vi "Video Playback.vi"() -> ()   [LabVIEW 2020, in "examples.lvlib"]
uses:
  examples.lvlib
  video_io/Reader/Reader.lvclass/Reader.ctl
  video_io/Reader/Reader.lvclass
  image/New Image (ARGB Preallocated).vi
  image/Size (ARGB).vi
  video_io/Reader/Set Frame Position (Index).vi
  video_io/Reader/Read Frame (ARGB Next).vi
  image/Draw Image to Picture (ARGB).vi
  video_io/Reader/Get Frame Position (Index).vi
  image/New Image (ARGB Preallocated).vi/3321fa97-f432-4e1e-8db9-a0df79aed21b.vi
  image/ARGB Colour to U32 Pixel Value.vi
  image/Size (ARGB).vi/69a1505b-b287-44ed-9ef9-f10ed7b260f4.vi
  video_io/Reader/Set Frame Position (Index).vi/acb2feee-aaa4-4f40-955f-c8ac8e9dff35.vi
  video_io/Reader/Read Frame (ARGB Next).vi/9eeb12df-7581-4bcd-a397-18dbd97d2298.vi
  image/Draw Image to Picture (ARGB).vi/8cd07b1b-062e-4fe4-9e87-2eb3dc89fe0e.vi
  video_io/Reader/Get Frame Position (Index).vi/acb2feee-aaa4-4f40-955f-c8ac8e9dff35.vi
  <vilib>/Utility/error.llb/Error Cluster From Error Code.vi
  image/image.lvlib
panel:
  out "File OK":bool
  in  "Play":bool
  in  "Video File":path
  in  "Position":u64(slide) scale=0.0..37.0
  out "Picture":picture
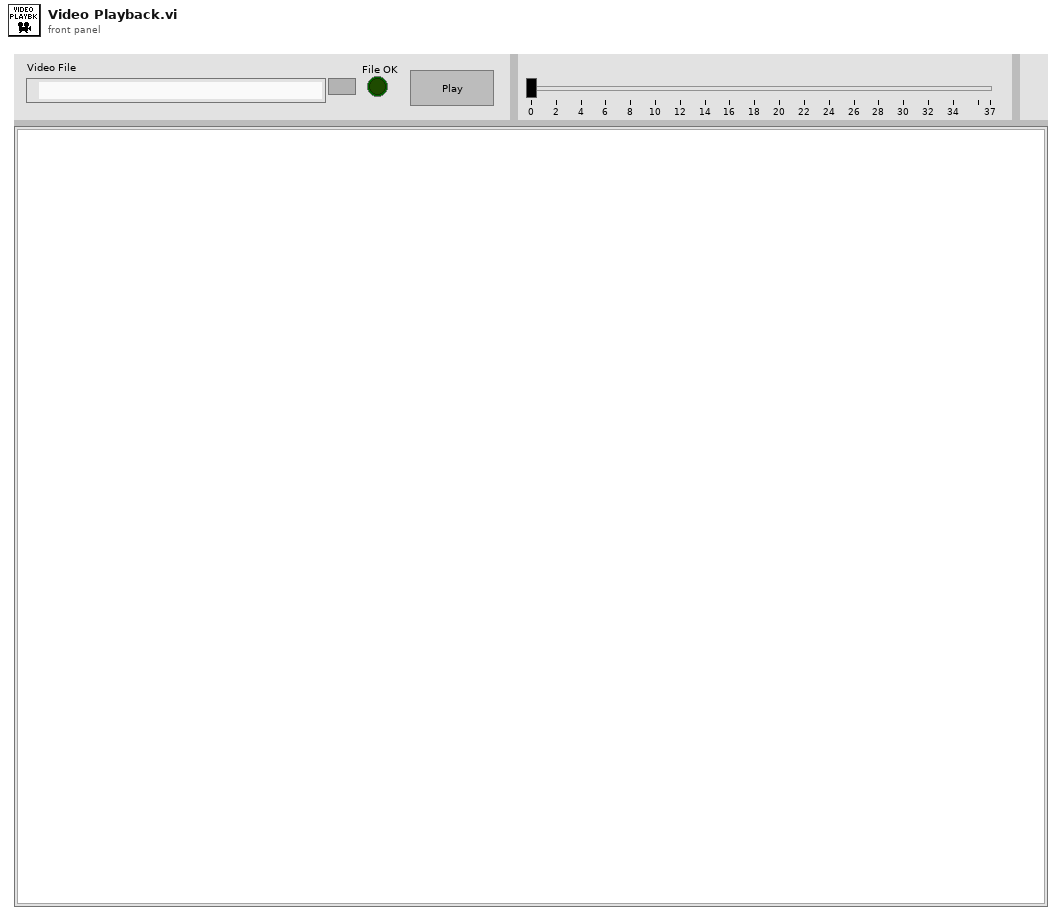
[diagram p1: front panel]
types:
  T1 = typedef "image.lvlib/ARGB Image.ctl" = refnum<data-value>
  T2 = enum8{"Enabled", "Disabled", "Disabled and Grayed Out"}
  T3 = typedef "common.lvlib/Image Size (Integer).ctl" = cluster{"Width":u16, "Height":u16}
  T4 = typedef "image.lvlib/Image Draw Offset.ctl" = cluster{"Left":i16, "Top":i16}
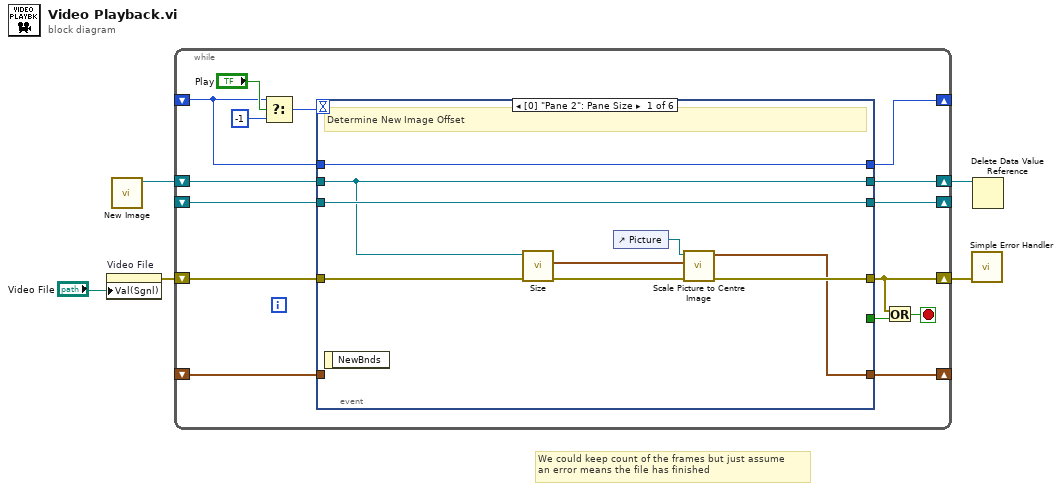
[diagram p0: block diagram]
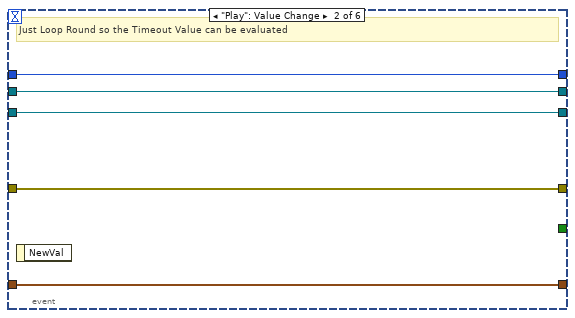
[diagram p2: hidden frame]
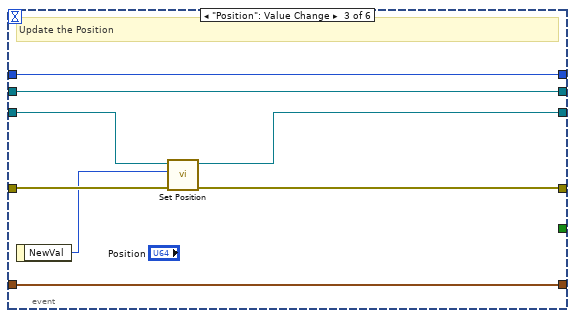
[diagram p3: hidden frame]
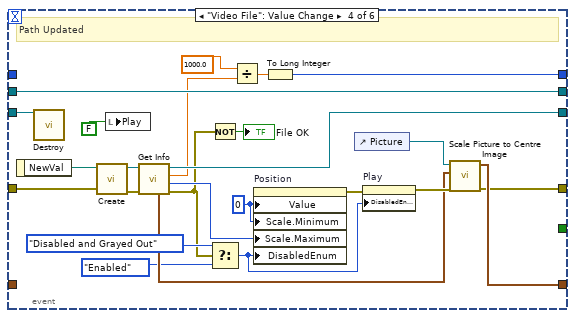
[diagram p4: hidden frame]
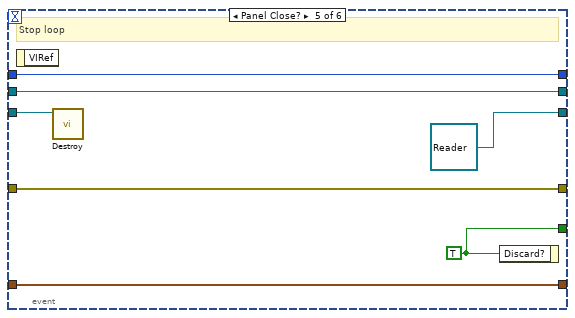
[diagram p5: hidden frame]
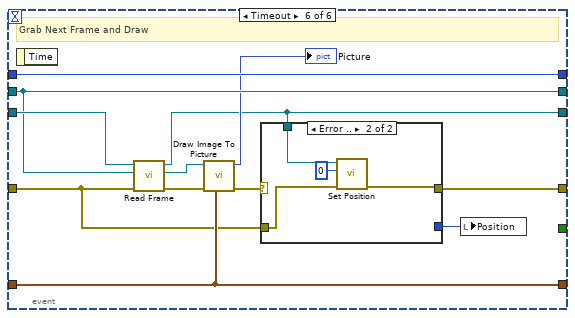
[diagram p6: hidden frame]
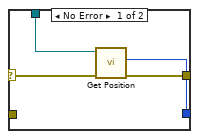
[diagram p7: hidden frame]
diagram:
  # "We could keep count of the frames but just assume\nan error means the file has finished"
  n1 = property on="Video File" class="Path"("Val(Sgnl)"="Video File") -> (error out=w1:errorcluster)  [unwired: 2 in, 1 out]
  n2 = call-poly "New Image.vi"() -> ("ARGB Image"=w5:T1)  [unwired: 10 in, 1 out]
  n3 = while {
    shift-right: [w17] -> w3
    shift-left: w5 -> [w19]
    shift-right: [w20] -> _
    shift-left: _ -> [w18]
    shift-right: [w16] -> _
    shift-left: _ -> [w12]
    shift-right: [w11] -> _
    shift-left: _ -> [w10]
    shift-right: [w8] -> w4
    shift-left: w1 -> [w9]
    stop <- w7 stop-if-true
    n4 = Select(t=w12, s="Play", f=-1) -> (s? t:f=w15:i32)
    n5 = event shown="[0] \"Pane 2\": Pane Size" {
      selector: _ -> [_ _ _ _ _ _]
      dyn-events: _ -> [_ _ _ _ _ _]
      timeout: w15 -> [_ _ _ _ _ _]
      tunnel: [w29 w30 w35 w65 refnum<class "Reader.lvclass"> refnum ("Reader") w78] -> w20
      tunnel: w19 -> [w24 w34 w42 w64 w70 w83]
      tunnel: w18 -> [w29 w30 w38 w46 w72 w84]
      tunnel: [w24 w34 w42 w64 w70 w83] -> w17
      tunnel: [w28 w33 w41 w60 w69 w86] -> w16
      tunnel: w12 -> [w28 w33 w41 _ w69 w86]
      tunnel: [w25 w32 w40 w53 w73 w80] -> w11
      tunnel: w10 -> [_ w32 w40 _ w73 w80]
      tunnel: [w26 w31 w36 w45 w71 w75] -> w8
      tunnel: w9 -> [w27 w31 w39 w54 w71 w76]
      tunnel: [_ _ _ _ w74 _] -> w6
      event Pane Size {
        # "Determine New Image Offset"
        n6 = event-data() -> ()  [unwired: 1 in, 1 out]
        n7 = call-poly "Size.vi"("error in (no error)"=w27, "ARGB Image in"=w24) -> ("error out"=w22:errorcluster, "Image Size"=w23:T3)  [unwired: 7 in, 1 out]
        n8 = control-ref of="Picture"() -> (w21:refnum<vi>)
        n9 = call "Scale Picture to Centre Image.vi"("error in (no error)"=w22, "Image Size"=w23, "Picture in"=w21) -> ("error out"=w26:errorcluster, "Draw Image to Picture Offset"=w25:T4)  [unwired: 6 in, 1 out]
      }
      event "Play": Value Change {
        # "Just Loop Round so the Timeout Value can be evaluated"
        n10 = event-data() -> ()  [unwired: 1 in, 1 out]
      }
      event "Position": Value Change {
        # "Update the Position"
        n11 = event-data() -> ("NewVal"=w37:u64)  [unwired: 1 in]
        n12 = call-poly "Set Position.vi"("error in (no error)"=w39, "Index"=w37, "Reader in"=w38) -> ("error out"=w36:errorcluster, "Reader"=w35:refnum<class "Reader.lvclass">)  [unwired: 7 in]
      }
      event "Video File": Value Change {
        w63 = u64 0 ("Position")
        # "Path Updated"
        n13 = event-data() -> ("NewVal"=w50:path)  [unwired: 1 in]
        n14 = call "Destroy.vi"("Reader in"=w46) -> ()  [unwired: 10 in, 1 out]
        n15 = call "Create.vi"("error in (no error)"=w54, "Path"=w50) -> ("error out"=w66:errorcluster, "Reader"=w67:refnum<class "Reader.lvclass">)  [unwired: 8 in]
        n16 = local write "Play"(FALSE ("Play")) -> ()
        n17 = call "Get Info.vi"("error in (no error)"=w66, "Reader in"=w67) -> ("error out"=w44:errorcluster, "Number of Frames"=w51:u64, "FPS"=w52:dbl, "Reader"=w65:refnum<class "Reader.lvclass">, "Size"=w57:T3)  [unwired: 5 in]
        n18 = Not(x=w44) -> (.not. x?=→"File OK":bool)
        n19 = Select(t=T2."Disabled and Grayed Out" ("Disabled"), s=w44, f=T2."Enabled" ("Disabled")) -> (s? t:f=w47:T2)
        n20 = Divide(x=1000.0, y=w52) -> (x/y=w61:dbl)
        n21 = property on="Position" class="Slide (strict)"("Value"=w63, "Scale.Minimum"=w63, "Scale.Maximum"=w51, "DisabledEnum"=w47) -> (error out=w59:errorcluster)  [unwired: 2 in, 1 out]
        n22 = To Long Integer(number=w61) -> (32bit integer=w60:i32)
        n23 = control-ref of="Picture"() -> (w56:refnum<vi>)
        n24 = property on="Play" class="Bool (strict)"(error in=w59, "DisabledEnum"=w47) -> (error out=w58:errorcluster)  [unwired: 1 in, 1 out]
        n25 = call "Scale Picture to Centre Image.vi"("error in (no error)"=w58, "Image Size"=w57, "Picture in"=w56) -> ("error out"=w45:errorcluster, "Draw Image to Picture Offset"=w53:T4)  [unwired: 6 in, 1 out]
      }
      event Panel Close? {
        w74 = TRUE ("Discard?")
        # "Stop loop"
        n26 = event-data() -> ()  [unwired: 1 in, 1 out]
        n27 = call "Destroy.vi"("Reader in"=w72) -> ()  [unwired: 10 in, 1 out]
        n28 = event-data("Discard?"=w74) -> ()  [unwired: 1 in, 1 out]
      }
      event Timeout {
        # "Grab Next Frame and Draw"
        n29 = event-data() -> ()  [unwired: 1 in, 1 out]
        n30 = call-poly "Read Frame.vi"("error in (no error)"=w76, "ARGB Image in"=w83, "Reader in"=w84) -> ("error out"=w82:errorcluster, "ARGB Image"=w85:T1, "Reader"=w78:refnum<class "Reader.lvclass">)  [unwired: 6 in]
        n31 = call-poly "Draw Image To Picture.vi"("Image Draw Offset (Default 0,0)"=w80, "error in (no error)"=w82, "ARGB Image Source in"=w85) -> ("error out"=w79:errorcluster, "Picture"=→"Picture":picture)  [unwired: 7 in]
        n32 = case shown="Error .." w79 {
          selector: w79 -> [w89 _]
          tunnel: [w88 w92] -> w75
          tunnel: w78 -> [w90 w94]
          tunnel: [w87 _] -> w77
          tunnel: w76 -> [_ w93]
          frame No Error {
            n33 = call-poly "Get Position.vi"("error in (no error)"=w89, "Reader in"=w90) -> ("error out"=w88:errorcluster, "Index"=w87:u64)  [unwired: 7 in, 1 out]
          }
          frame Error {
            n34 = call-poly "Set Position.vi"("error in (no error)"=w93, "Index"=u64 0, "Reader in"=w94) -> ("error out"=w92:errorcluster)  [unwired: 7 in, 1 out]
          }
        }
        n35 = local write "Position"(w77) -> ()
      }
    }
    n36 = Or(x=w8, y=w6) -> (x .or. y?=w7:bool)
  }
  n37 = call <vilib>:"Simple Error Handler.vi"("error in (no error)"=w4) -> ()  [unwired: 4 in, 5 out]
  n38 = Delete Data Value Reference(data value reference=w3) -> ()  [unwired: 1 in, 2 out]
